vi "Lube Program C (SubVI).vi"(0 "References":T1, 7 "Strain Input":T2={"cDAQ Chassis"=1, "9237 Slot"=5, "Signals"=[0.0, 0.0, 0.0, 0.0]}, 11 "Enable":bool) -> (15 "Error":errorcluster)   [LabVIEW 2010]
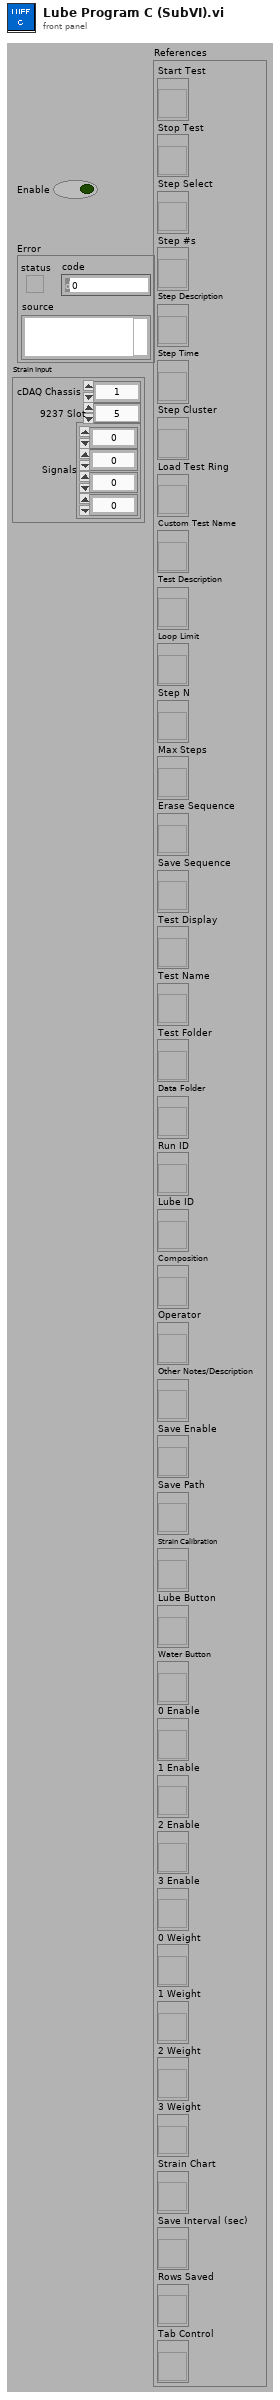
[diagram p1: front panel]
types:
  T1 = cluster{"Start Test":refnum<vi>, "Stop Test":refnum<vi>, "Step Select":refnum<vi>, "Step #s":refnum<vi>, "Step Description":refnum<vi>, "Step Time":refnum<vi>, "Step Cluster":refnum<vi>, "Load Test Ring":refnum<vi>, "Custom Test Name":refnum<vi>, "Test Description":refnum<vi>, "Loop Limit":refnum<vi>, "Step N":refnum<vi>, "Max Steps":refnum<vi>, "Erase Sequence":refnum<vi>, "Save Sequence":refnum<vi>, "Test Display":refnum<vi>, "Test Name":refnum<vi>, "Test Folder":refnum<vi>, "Data Folder":refnum<vi>, "Run ID":refnum<vi>, "Lube ID":refnum<vi>, "Composition":refnum<vi>, "Operator":refnum<vi>, "Other Notes/Description":refnum<vi>, "Save Enable":refnum<vi>, "Save Path":refnum<vi>, "Strain Calibration":refnum<vi>, "Lube Button":refnum<vi>, "Water Button":refnum<vi>, "0 Enable":refnum<vi>, "1 Enable":refnum<vi>, "2 Enable":refnum<vi>, "3 Enable":refnum<vi>, "0 Weight":refnum<vi>, "1 Weight":refnum<vi>, "2 Weight":refnum<vi>, "3 Weight":refnum<vi>, "Strain Chart":refnum<vi>, "Save Interval (sec)":refnum<vi>, "Rows Saved":refnum<vi>, "Tab Control":refnum<vi>}
  T2 = cluster{"cDAQ Chassis":i32, "9237 Slot":i32, "Signals":dbl[]}
  T3 = enum8{"Enabled", "Disabled", "Disabled and Grayed Out"}
  T4 = cluster{"Output Values":dbl[], "Linear Equations":string[][], "COF Values":dbl[], "Signals":dbl[]}
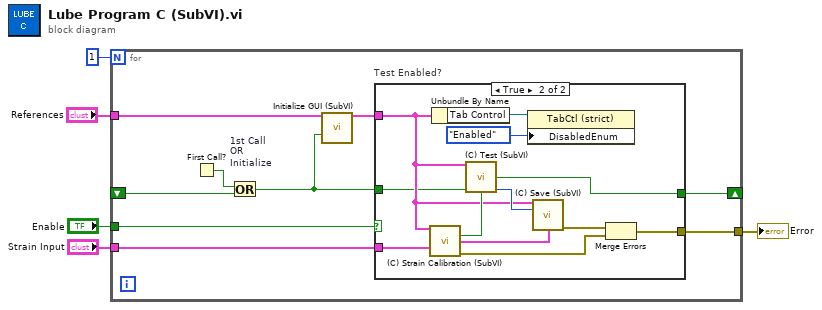
[diagram p0: block diagram]
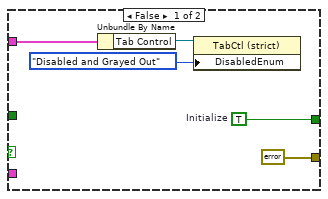
[diagram p2: hidden frame]
diagram:
  n1 = for {
    N: 1 -> [_]
    tunnel: "References" -> [w13]
    shift-right: [w12] -> _
    shift-left: _ -> [w7]
    tunnel: [w10] -> w5
    tunnel: "Strain Input" -> [w9]
    tunnel: "Enable" -> [w8]
    n2 = First Call?() -> (First Call?: T/F=w11:bool)
    n3 = Or "1st Call\nOR\nInitialize"(x=w11, y=w7) -> (x .or. y?=w6:bool)
    n4 = call "Initialize GUI (SubVI).vi"("References IN"=w13, "Initialize Command"=w6) -> ("References OUT"=w14:T1)  [unwired: 13 in]
    n5 = case "Test Enabled?" shown="True" w8 {
      tunnel: w14 -> [w18 w22]
      tunnel: [w15 w21] -> w12
      tunnel: [errorcluster {"status"=FALSE, "code"=0, "source"=""} w26] -> w10
      tunnel: w9 -> [_ w25]
      tunnel: w6 -> [_ w20]
      frame False {
        w15 = TRUE  # Initialize
        n6 = Unbundle By Name(w18) -> ("Tab Control"=w17:refnum<vi>)
        n7 = property class="TabCtl (strict)"(reference=w17, "DisabledEnum"=T3."Disabled and Grayed Out" ("Disabled")) -> ()  [unwired: 1 in, 2 out]
      }
      frame True {
        n8 = call "(C) Strain Calibration (SubVI).vi"("References"=w22, "Strain Input"=w25) -> ("Strain OK?"=w27:bool, "Strain Values"=w31:T4, "Calibration Error"=w28:errorcluster)  [unwired: 11 in]
        n9 = Unbundle By Name(w22) -> ("Tab Control"=w23:refnum<vi>)
        n10 = call "(C) Test (SubVI).vi"("References IN"=w22, "Initialize"=w20, "Strain OK?"=w27) -> ("STOP-PROGRAM"=w21:bool, "Step Number"=w30:i32)  [unwired: 11 in]
        n11 = property class="TabCtl (strict)"(reference=w23, "DisabledEnum"=T3."Enabled" ("Disabled")) -> ()  [unwired: 1 in, 2 out]
        n12 = call "(C) Save (SubVI).vi"("References"=w22, "Step Number"=w30, "Strain Values"=w31) -> ("Save Error"=w29:errorcluster)  [unwired: 12 in]
        n13 = Merge Errors(w29, w28) -> (w26:errorcluster)
      }
    }
  }
  "Error" <- w5
